vi "5.3-Forebrain Mapper.vi"() -> ()   [LabVIEW 2010]
uses:
  5.0-Global.vi
  <vilib>/robotics/Navigation/shared/WorldMap/OccupancyGridWorldMap/NI_Robotics_OccupancyGridWorldMap.lvclass
panel:
  out "Intensity Graph":dbl[][](graph)
  out "XY Graph":cluster{dbl[], dbl[]}(graph)
  out "Heartbeat":bool
  in  "Boolean":bool
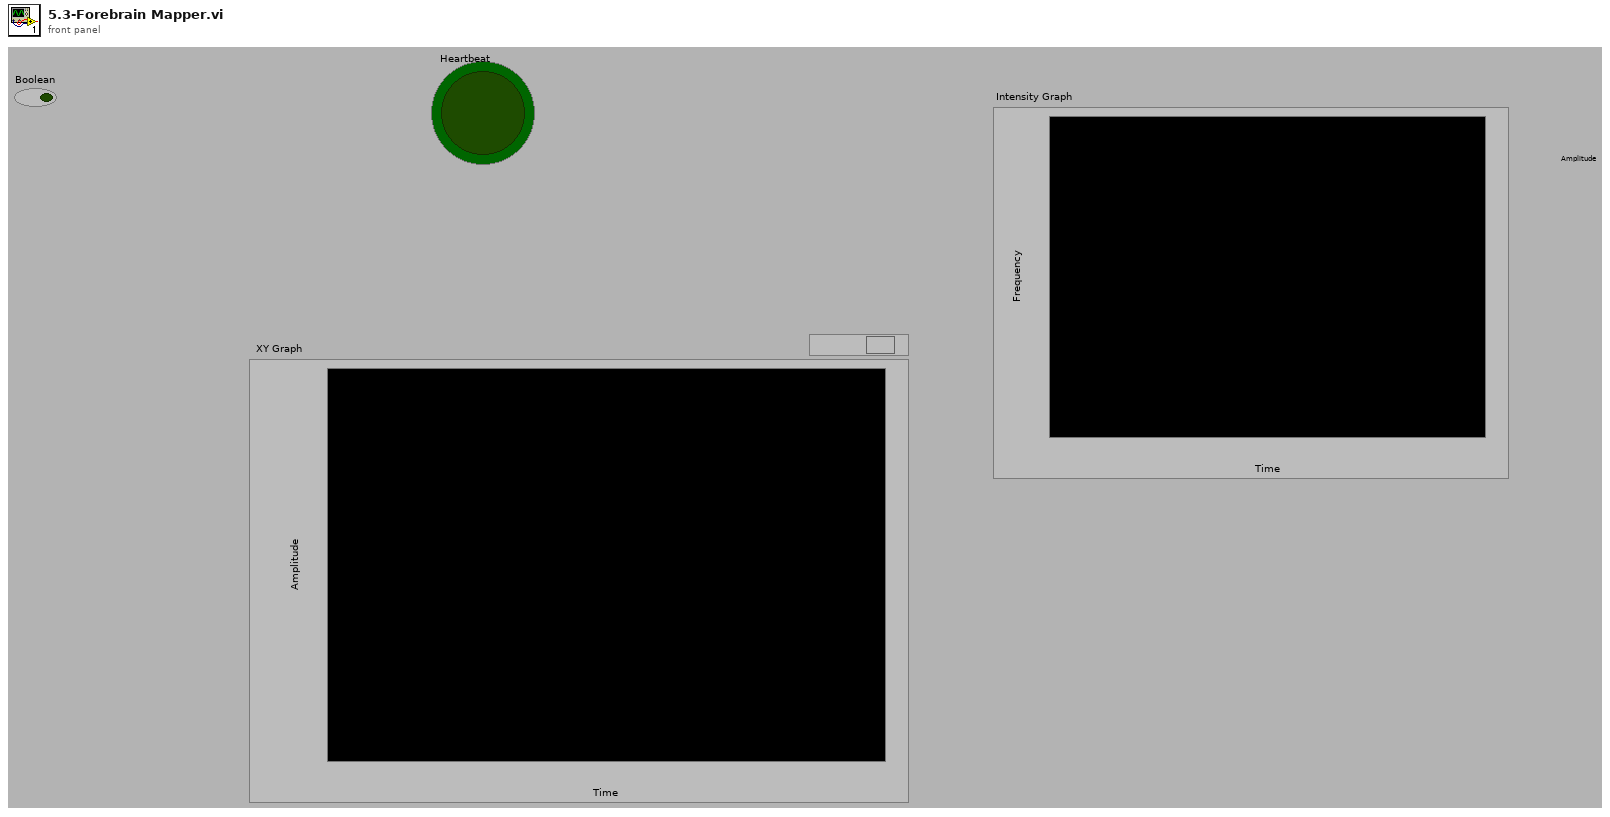
[diagram p1: front panel]
types:
  T1 = typedef "MDF XY.ctl" = cluster{"Waypoint #":dbl, "X (waypoint)":ext, "Y  (waypoint)":ext}
  T2 = cluster{"X (Current)":dbl, "Y (Current) ":dbl, "Heading":dbl, "Steering Angle":dbl}
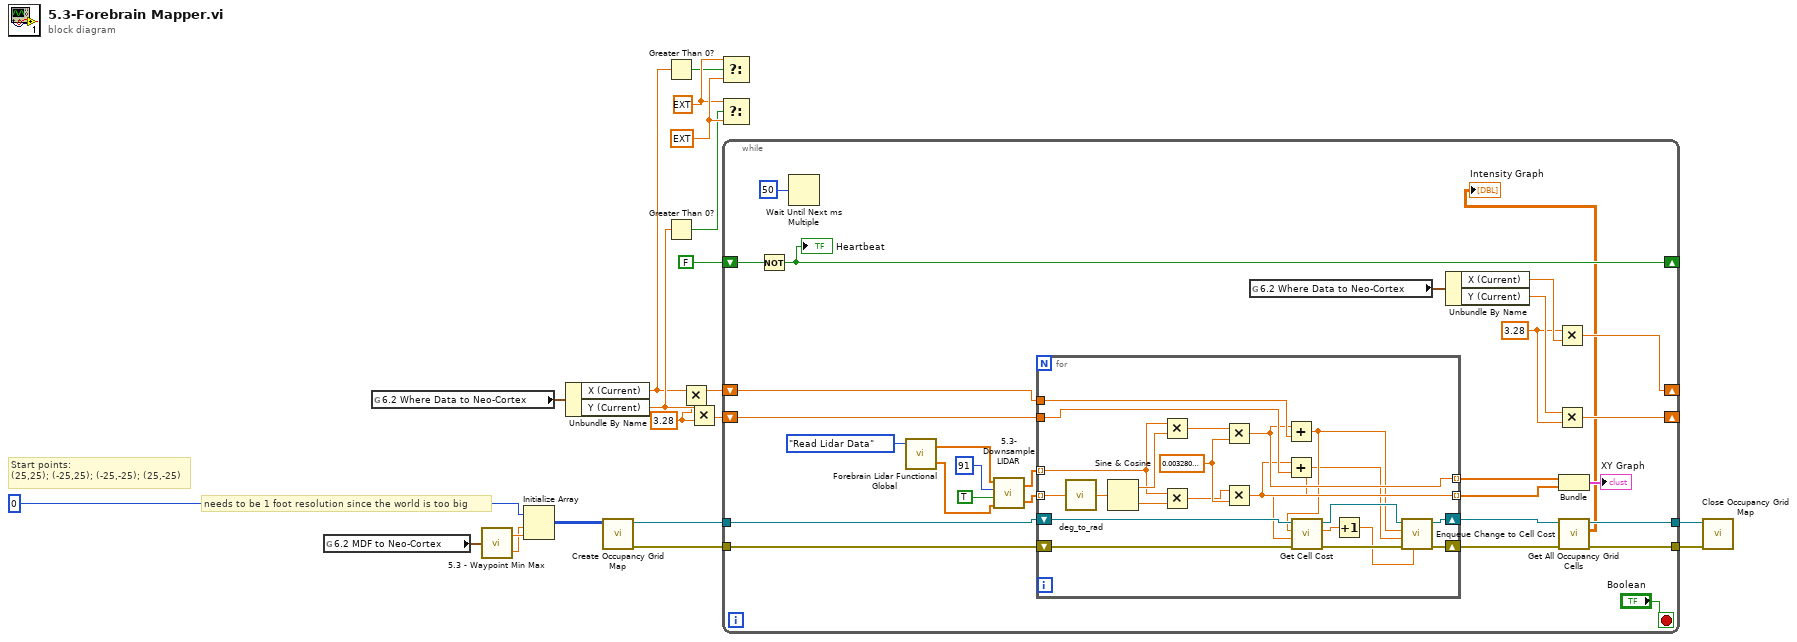
[diagram p0: block diagram]
diagram:
  w1 = 3.28 ("y")
  w15 = ext -25.0 ("element")
  w14 = ext 25.0 ("element")
  # "Start points:\n(25,25); (-25,25); (-25,-25); (25,-25)"
  # "needs to be 1 foot resolution since the world is too big"
  n1 = global read "5.0-Global.vi" "6.2 MDF to Neo-Cortex"() -> (w19:T1[])
  n2 = global read "5.0-Global.vi" "6.2 Where Data to Neo-Cortex"() -> (w16:T2)
  n3 = call "5.3 - Waypoint Min Max.vi"("6.2 MDF to Neo-Cortex"=w19) -> ("Y Dimension (Row)"=w17:ext, "X Dimension (Column)"=w18:ext)
  n4 = Initialize Array(u32 0 ("element"), w17, w18) -> (w10:u32[][])
  n5 = Unbundle By Name(w16) -> ("X (Current)"=w4:dbl, "Y (Current)"=w5:dbl)
  n6 = call <vilib>:"Create Occupancy Grid Map.vi"("occupancy grid"=w10) -> ("error out"=w6:errorcluster, "map reference out"=w9:refnum<data-value>)  [unwired: 9 in]
  n7 = Greater Than 0?(x=w4) -> (x > 0?=w12:bool)
  n8 = Greater Than 0?(x=w5) -> (x > 0?=w13:bool)
  n9 = Multiply(x=w4, y=w1) -> (x*y=w3:dbl)
  n10 = Multiply(x=w5, y=w1) -> (x*y=w2:dbl)
  n11 = Select(t=w14, s=w12, f=w15) -> ()  [unwired: 1 out]
  n12 = Select(t=w14, s=w13, f=w15) -> ()  [unwired: 1 out]
  n13 = while {
    shift-right: [w35] -> _
    shift-left: w3 -> [w42]
    shift-right: [w34] -> _
    shift-left: w2 -> [w41]
    shift-right: [w31] -> _
    shift-left: FALSE -> [w32]
    tunnel: w9 -> [w27]
    tunnel: [w25] -> w8
    tunnel: [w24] -> w7
    tunnel: w6 -> [w26]
    stop <- "Boolean" stop-if-true
    w33 = 3.28 ("y")
    n14 = Not(x=w32) -> (.not. x?=w31:bool)
    "Heartbeat" <- w31
    n15 = Wait Until Next ms Multiple(millisecond multiple=u32 50) -> ()  [unwired: 1 out]
    n16 = call "Forebrain Lidar Functional Global.vi"("Lidar Action"=enum16{"Set Lidar Data", "Read Lidar Data"}."Read Lidar Data") -> ("Lidar Angle Data Out (Degrees)"=w47:sgl[], "Lidar Magnitude Data Out (mm)"=w48:sgl[])  [unwired: 2 in]
    n17 = call "5.3- Downsample LIDAR.vi"("Corresponding Input Array For Minimum"=w47, "Minimum?"=TRUE, "Numeric"=91, "Input Array"=w48) -> ("Corresponding Output Array only for Minimum"=w44:sgl[], "Output Array"=w43:sgl[])
    n18 = for {
      tunnel: w44 -> [w71] mode=indexing
      tunnel: w43 -> [w62] mode=indexing
      tunnel: w42 -> [w67]
      tunnel: w41 -> [w66]
      tunnel: [w55] -> w30 mode=indexing
      tunnel: [w54] -> w29 mode=indexing
      shift-right: [w57] -> w22
      shift-left: w27 -> [w58]
      shift-right: [w53] -> w23
      shift-left: w26 -> [w52]
      w68 = sgl 0.00328 ("y")
      n19 = call "deg_to_rad.vi"("Degrees"=w71) -> ("Radians"=w65:dbl)
      n20 = Sine & Cosine(0:w65) -> (1:w69:dbl, 2:w70:dbl)
      n21 = Multiply(x=w62, y=w69) -> (x*y=w64:dbl)
      n22 = Multiply(x=w62, y=w70) -> (x*y=w63:dbl)
      n23 = Multiply(x=w64, y=w68) -> (x*y=w55:dbl)
      n24 = Multiply(x=w63, y=w68) -> (x*y=w54:dbl)
      n25 = Add(x=w55, y=w67) -> (x+y=w51:dbl)
      n26 = Add(x=w54, y=w66) -> (x+y=w50:dbl)
      n27 = call <vilib>:"Get Cell Cost.vi"("error in (no error)"=w52, "y"=w50, "x"=w51, "map reference in"=w58) -> ("error out"=w61:errorcluster, "cost"=w60:dbl, "map reference out"=w59:refnum<data-value>)  [unwired: 4 in, 1 out]
      n28 = Increment(x=w60) -> (x+1=w56:dbl)
      n29 = call <vilib>:"Enqueue Change to Cell Cost.vi"("cost"=w56, "error in (no error)"=w61, "y"=w50, "x"=w51, "map reference in"=w59) -> ("error out"=w53:errorcluster, "map reference out"=w57:refnum<data-value>)  [unwired: 5 in]
    }
    n30 = global read "5.0-Global.vi" "6.2 Where Data to Neo-Cortex"() -> (w40:T2)
    n31 = Unbundle By Name(w40) -> ("X (Current)"=w38:dbl, "Y (Current)"=w39:dbl)
    n32 = Multiply(x=w33, y=w38) -> (x*y=w35:dbl)
    n33 = Multiply(x=w39, y=w33) -> (x*y=w34:dbl)
    n34 = Bundle(w30, w29) -> (→"XY Graph":cluster{dbl[], dbl[]})  [unwired: 1 in]
    n35 = call <vilib>:"Get All Occupancy Grid Cells.vi"("error in (no error)"=w23, "map reference in"=w22) -> ("error out"=w24:errorcluster, "occupancy grid"=→"Intensity Graph":dbl[][], "map reference out"=w25:refnum<data-value>)  [unwired: 7 in]
  }
  n36 = call <vilib>:"Close Occupancy Grid Map.vi"("error in (no error)"=w7, "map reference in"=w8) -> ()  [unwired: 9 in, 1 out]
